vi "Deploy with Reboot and Retry.vi"(8 "error in":errorcluster, 10 "System Definition File":path, 11 "VeriStand Test Case in":refnum<class "VeriStandTestCase.lvclass">) -> (0 "error out":errorcluster, 3 "VeriStand Test Case out":refnum<class "VeriStandTestCase.lvclass">)   [LabVIEW 2019, in "cRIO System Tests.lvclass"]
uses:
  cRIO System Tests.lvclass
  <vilib>/NI/VeriStand Custom Device Testing Tools/VeriStandTestCase/VeriStandTestCase.lvclass
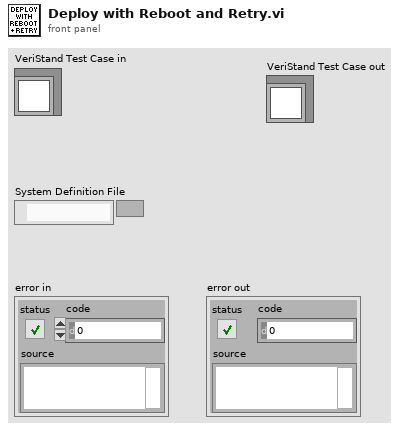
[diagram p1: front panel]
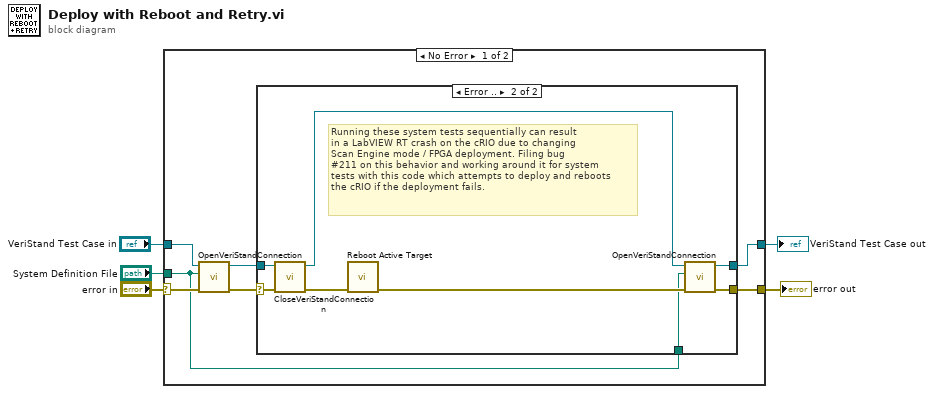
[diagram p0: block diagram]
diagram:
  n1 = case shown="No Error" "error in" {
    selector: "error in" -> [w9 w24]
    tunnel: [w12 w23] -> w1
    tunnel: [w10 w24] -> w5
    tunnel: "System Definition File" -> [w8 _]
    tunnel: "VeriStand Test Case in" -> [w6 w23]
    frame No Error {
      n2 = call-dynamic "OpenVeriStandConnection.vi"("error in (no error)"=w9, "System Definition File"=w8, "VeriStand Test Case in"=w6) -> ("error out"=w7:errorcluster, "VeriStand Test Case out"=w11:refnum<class "VeriStandTestCase.lvclass">)  [unwired: 6 in, 1 out]
      n3 = case shown="Error .." w7 {
        selector: w7 -> [w14 w21]
        tunnel: [w14 w17] -> w10
        tunnel: w11 -> [w13 w22]
        tunnel: [w13 w19] -> w12
        tunnel: w8 -> [_ w15]
        frame No Error {
        }
        frame Error {
          # "Running these system tests sequentially can result\nin a LabVIEW RT crash on the cRIO due to changing\nScan Engine mode / FPGA deployment. Filing bug\n#211 on this behavior and working around it for system\ntests with this code which attempts to deploy and reboots\nthe cRIO if the deployment fails."
          n4 = call-dynamic "CloseVeriStandConnection.vi"("error in (no error)"=w21, "VeriStand Test Case in"=w22) -> ("error out"=w16:errorcluster, "VeriStand Test Case out"=w20:refnum<class "VeriStandTestCase.lvclass">)  [unwired: 8 in]
          n5 = call "Reboot Active Target.vi"("error in"=w16) -> ("error out"=w18:errorcluster)  [unwired: 10 in]
          n6 = call-dynamic "OpenVeriStandConnection.vi"("error in (no error)"=w18, "System Definition File"=w15, "VeriStand Test Case in"=w20) -> ("error out"=w17:errorcluster, "VeriStand Test Case out"=w19:refnum<class "VeriStandTestCase.lvclass">)  [unwired: 6 in, 1 out]
        }
      }
    }
    frame Error {
    }
  }
  "error out" <- w5
  "VeriStand Test Case out" <- w1
